vi "Draw.vi"(8 "error in":errorcluster, 11 "GoL in":refnum<class "GoL.lvclass">) -> (0 "error out":errorcluster, 2 "2D Picture":picture, 3 "GoL out":refnum<class "GoL.lvclass">)   [LabVIEW 2026, in "GoL.lvlib" / "GoL.lvclass"]
uses:
  GoL.lvclass
  GoL.lvclass/GoL.ctl
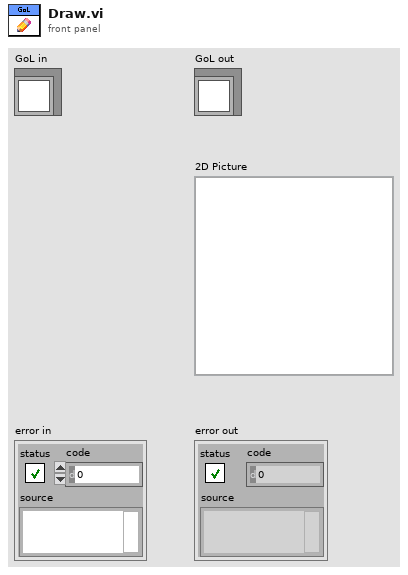
[diagram p1: front panel]
types:
  T1 = cluster{"left":i16, "top":i16, "right":i16, "bottom":i16}
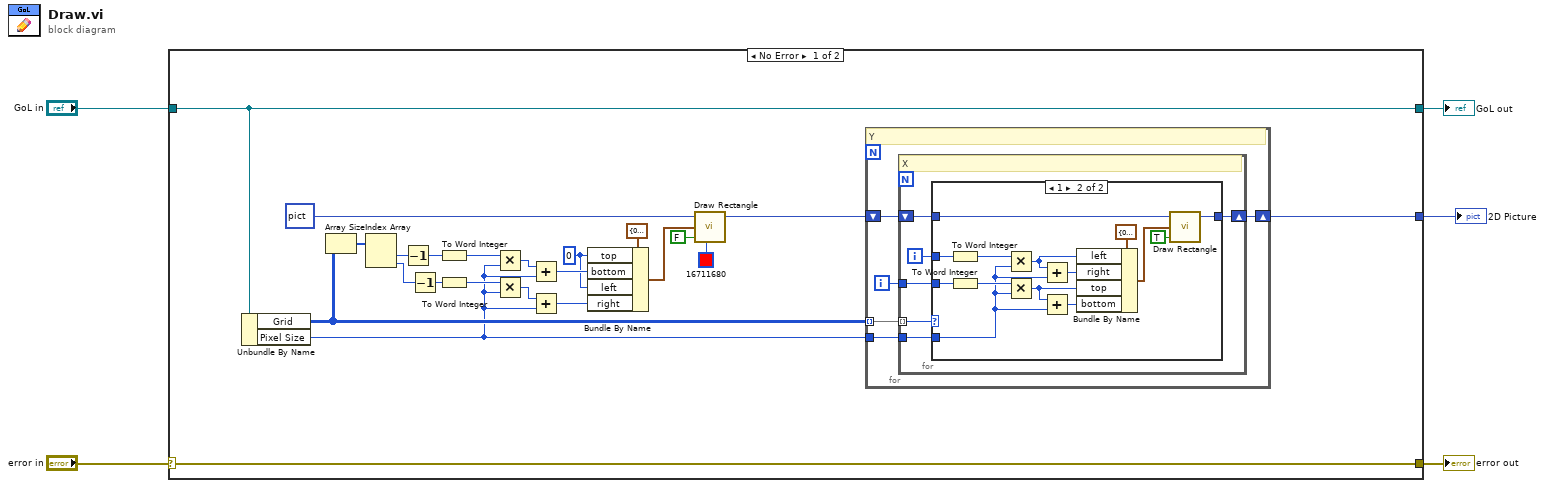
[diagram p0: block diagram]
diagram:
  n1 = case shown="No Error" "error in" {
    selector: "error in" -> [w28 w56]
    tunnel: [w28 w56] -> w4
    tunnel: [w27 w55] -> w2
    tunnel: "GoL in" -> [w27 w55]
    tunnel: [w26 _] -> w1
    frame No Error {
      w10 = i16 0 ("top")
      n2 = Unbundle By Name(w27) -> ("Grid"=w25:u8[][], "Pixel Size"=w19:i16)
      n3 = Array Size(array=w25) -> (size(s)=w23:i32[])
      n4 = Index Array(array=w23) -> (element #1=w9:i32, element #2=w8:i32)  [unwired: 2 in]
      n5 = Decrement(x=w9) -> (x-1=w7:i32)
      n6 = Decrement(x=w8) -> (x-1=w6:i32)
      n7 = To Word Integer(number=w7) -> (16bit integer=w20:i16)
      n8 = To Word Integer(number=w6) -> (16bit integer=w21:i16)
      n9 = Multiply(x=w20, y=w19) -> (x*y=w17:i16)
      n10 = Multiply(x=w21, y=w19) -> (x*y=w16:i16)
      n11 = Add(x=w17, y=w19) -> (x+y=w18:i16)
      n12 = Add(x=w16, y=w19) -> (x+y=w15:i16)
      n13 = Bundle By Name(cluster=T1 {"left"=0, "top"=0, "right"=0, "bottom"=0} ("rect"), "top"=w10, "bottom"=w18, "left"=w10, "right"=w15) -> (w14:T1)
      n14 = call <vilib>:"Draw Rectangle.vi"("picture"=picture data[5B] ("new picture"), "rect"=w14, "fill?(F)"=FALSE, "color(black)"=u32 16711680) -> ("new picture"=w11:picture)  [unwired: 5 in]
      n15 = for {
        tunnel: w25 -> [w33] mode=indexing
        tunnel: w19 -> [w32]
        shift-right: [w31] -> w26
        shift-left: w11 -> [w30]
        i -> [w29]
        # "Y"
        n16 = for {
          tunnel: w33 -> [w39] mode=indexing
          tunnel: w32 -> [w37]
          shift-right: [w36] -> w31
          shift-left: w30 -> [w35]
          tunnel: w29 -> [w34]
          i -> [w38]
          # "X"
          n17 = case shown="1" w39 {
            tunnel: w38 -> [_ w53]
            tunnel: w37 -> [_ w42]
            tunnel: [w40 w52] -> w36
            tunnel: w35 -> [w40 w51]
            tunnel: w34 -> [_ w45]
            frame Default {
            }
            frame 1 {
              n18 = To Word Integer(number=w53) -> (16bit integer=w43:i16)
              n19 = To Word Integer(number=w45) -> (16bit integer=w44:i16)
              n20 = Multiply(x=w43, y=w42) -> (x*y=w49:i16)
              n21 = Multiply(x=w44, y=w42) -> (x*y=w47:i16)
              n22 = Add(x=w49, y=w42) -> (x+y=w48:i16)
              n23 = Add(x=w47, y=w42) -> (x+y=w46:i16)
              n24 = Bundle By Name(cluster=T1 {"left"=0, "top"=0, "right"=0, "bottom"=0} ("rect"), "left"=w49, "right"=w48, "top"=w47, "bottom"=w46) -> (w50:T1)
              n25 = call <vilib>:"Draw Rectangle.vi"("picture"=w51, "rect"=w50, "fill?(F)"=TRUE) -> ("new picture"=w52:picture)  [unwired: 6 in]
            }
          }
        }
      }
    }
    frame Error {
    }
  }
  "error out" <- w4
  "GoL out" <- w2
  "2D Picture" <- w1
